vi "GetTypeOfTest.vi"(8 "error in (no error)":errorcluster, 10 "VI Refnum":refnum<vi>) -> (0 "error out":errorcluster, 2 "Type":T1)   [LabVIEW 2019, in "LVUnitTestBuilder.lvclass"]
doc: "Gets the type of test from the specified VI Refnum."
uses:
  LVUnitTestBuilder.lvclass
  Type.ctl
  <vilib>/addons/analyzer/_analyzerutils.llb/VIAnUtil Check Type If ErrClust.vi
  <vilib>/Utility/Data Type/NI_Data Type.lvlib
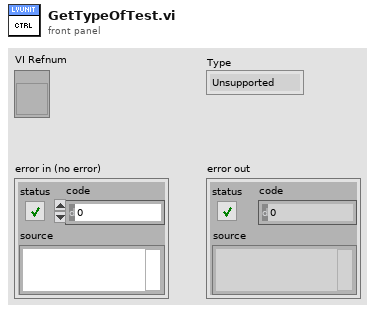
[diagram p1: front panel]
types:
  T1 = typedef "LVUnitTestBuilder.lvclass/Type.ctl" = enum16{"Unsupported", "Fact", "Theory"}
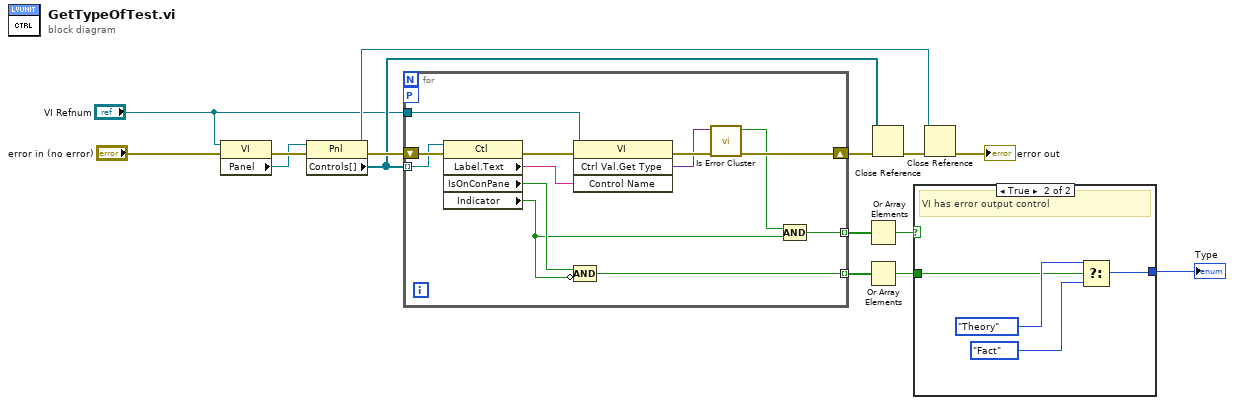
[diagram p0: block diagram]
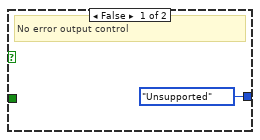
[diagram p2: hidden frame]
diagram:
  n1 = property class="VI"(reference="VI Refnum", error in="error in (no error)") -> (error out=w15:errorcluster, "Panel"=w14:refnum<vi>)  [unwired: 1 out]
  n2 = property class="Pnl"(reference=w14, error in=w15) -> (reference out=w12:refnum<vi>, error out=w13:errorcluster, "Controls[]"=w9:refnum<vi>[])
  n3 = for {
    tunnel: w9 -> [w26] mode=indexing
    shift-right: [w20] -> w11
    shift-left: w13 -> [w27]
    tunnel: [w28] -> w7 mode=indexing
    workers-P: _ -> [_]
    tunnel: "VI Refnum" -> [w23]
    tunnel: [w16] -> w3 mode=indexing
    n4 = property class="Ctl"(reference=w26, error in=w27) -> (error out=w24:errorcluster, "Label.Text"=w22:string, "IsOnConPane"=w25:bool, "Indicator"=w17:bool)  [unwired: 1 out]
    n5 = invoke class="VI" method="Ctrl Val.Get Type"(reference=w23, error in=w24, "Control Name"=w22) -> (error out=w21:errorcluster, "Ctrl Val.Get Type"=w19:variant)  [unwired: 1 in, 2 out]
    n6 = Compound Arithmetic op=AND(w25, invert w17) -> (w28:bool)
    n7 = call <vilib>:"Is Error Cluster.vi"("error in (no error)"=w21, "variant"=w19) -> ("error out"=w20:errorcluster, "is error cluster?"=w18:bool)  [unwired: 8 in]
    n8 = Compound Arithmetic op=AND(w18, w17) -> (w16:bool)
  }
  n9 = Or Array Elements(Boolean array=w3) -> (logical OR=w2:bool)
  n10 = Or Array Elements(Boolean array=w7) -> (logical OR=w1:bool)
  n11 = Close Reference(reference=w9, error in (no error)=w11) -> (error out=w10:errorcluster)
  n12 = case shown="True" w2 {
    tunnel: [Type."Unsupported" ("Type") w33] -> w5
    tunnel: w1 -> [_ w30]
    frame False {
      # "No error output control"
    }
    frame True {
      # "VI has error output control"
      n13 = Select(t=Type."Theory" ("Type"), s=w30, f=Type."Fact" ("Type")) -> (s? t:f=w33:T1)
    }
  }
  "Type" <- w5
  n14 = Close Reference(reference=w12, error in (no error)=w10) -> (error out=→"error out":errorcluster)
